vi "Try Match Response.vi"(8 "error in":errorcluster, 10 "ICAN CC Frame":refnum<class "ICAN CC Frame.lvclass">, 11 "Block Upload End Transfer in":refnum<class "Block Upload End Transfer.lvclass">) -> (0 "error out":errorcluster, 2 "Match":bool, 3 "SDO Transfer out":refnum<class "SDO Transfer.lvclass">)   [LabVIEW 2020, in "CANopen.lvlib" / "SDO Manager.lvlib" / "Block Upload End Transfer.lvclass"]
uses:
  Block Upload End Transfer.lvclass
  SDO Transfer/SDO Transfer.lvclass
  HAL/Source/Interfaces/ICAN CC Frame/ICAN CC Frame.lvclass
  Block Upload End Transfer.lvclass/Block Upload End Transfer.ctl
  CANopen Message/CANopen Message.lvclass
  SDO Transfer/SDO abort code.ctl
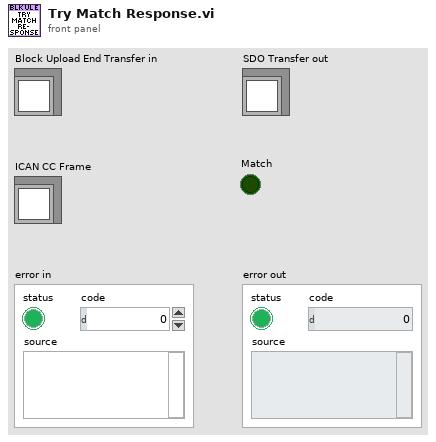
[diagram p1: front panel]
types:
  T1 = typedef "CANopen.lvlib/SDO Manager.lvlib/SDO Transfer.lvclass/SDO abort code.ctl" = u32
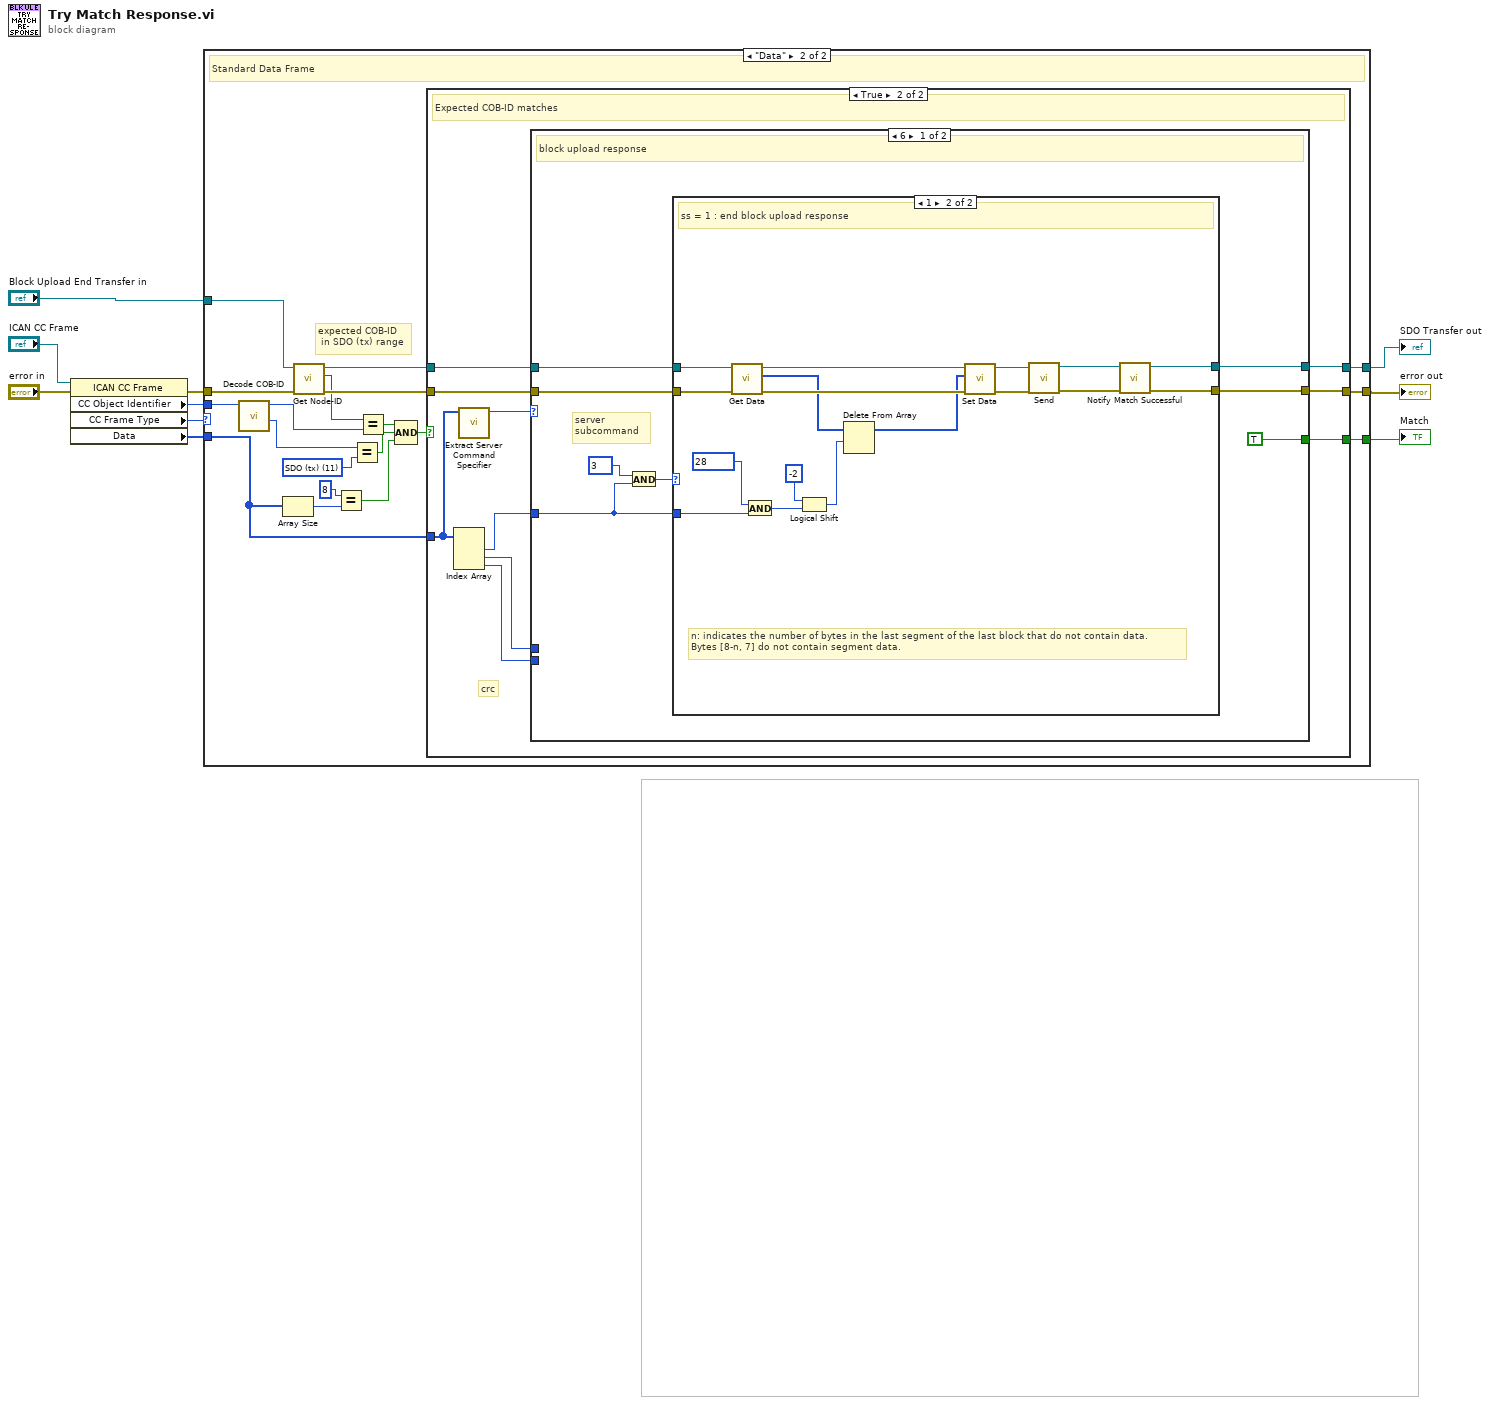
[diagram p0: block diagram]
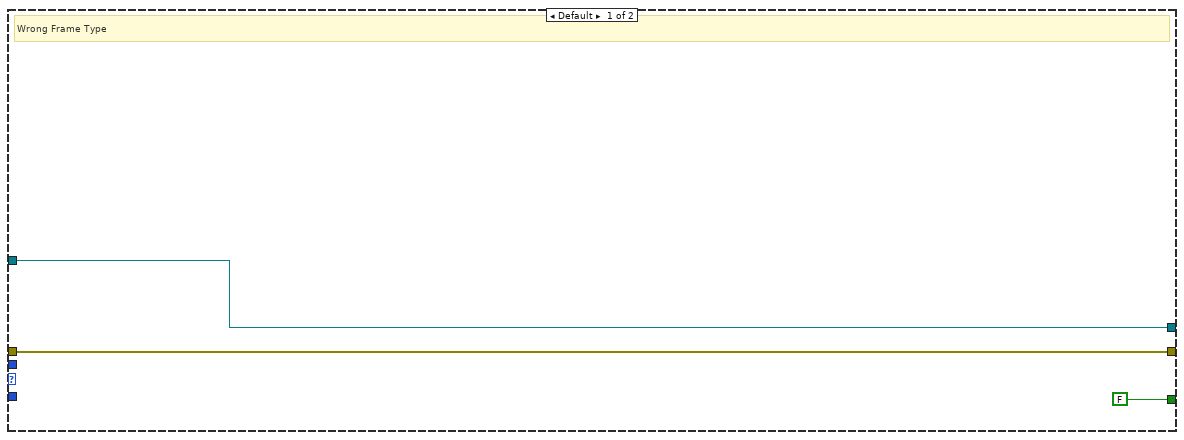
[diagram p2: hidden frame]
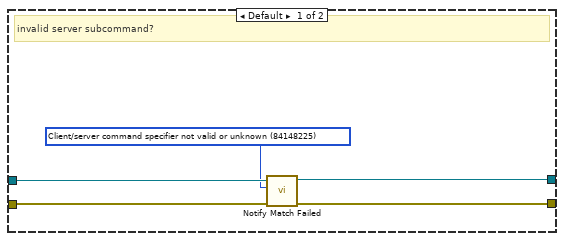
[diagram p4: hidden frame]
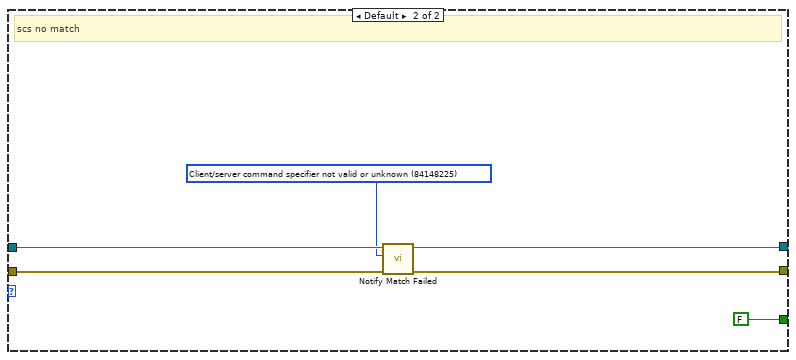
[diagram p5: hidden frame]
diagram:
  n1 = property class="ICAN CC Frame"(reference="ICAN CC Frame", error in="error in") -> (error out=w10:errorcluster, "CC Object Identifier"=w9:u32, "CC Frame Type"=w7:enum8{"Data", "Remote", "Error", "Overload"}, "Data"=w8:u8[])  [unwired: 1 out]
  n2 = case shown="\"Data\"" w7 {
    tunnel: w10 -> [w12 w32]
    tunnel: "Block Upload End Transfer in" -> [w11 w31]
    tunnel: [w11 w28] -> w4
    tunnel: [w12 w27] -> w6
    tunnel: [FALSE w26] -> w5
    tunnel: w9 -> [_ w25]
    tunnel: w8 -> [_ w14]
    frame Default {
      # "Wrong Frame Type"
    }
    frame "Data" {
      w22 = u8 11 items=["NMT"=0, "EMCY/SYNC"=1, "TIME"=2, "PDO1 (tx)"=3, "PDO1 (rx)"=4, "PDO2 (tx)"=5, "PDO2 (rx)"=6, "PDO3 (tx)"=7, "PDO3 (rx)"=8, "PDO4 (tx)"=9, "PDO4 (rx)"=10, "SDO (tx)"=11, "SDO (rx)"=12, "NMT error control"=14] ("Function Code")
      # "expected COB-ID\n in SDO (tx) range"
      # "Standard Data Frame"
      n3 = call "Decode COB-ID.vi"("COD-ID"=w25) -> ("Function Code"=w21:u8, "Node-ID"=w24:u8)  [unwired: 9 in]
      n4 = Array Size(array=w14) -> (size(s)=w20:i32)
      n5 = call "Get Node-ID.vi"("error in"=w32, "SDO Transfer in"=w31) -> ("error out"=w29:errorcluster, "Node-ID"=w23:u8, "SDO Transfer out"=w30:refnum<class "Block Upload End Transfer.lvclass">)  [unwired: 7 in]
      n6 = Equal?(x=8, y=w20) -> (x = y?=w15:bool)
      n7 = Equal?(x=w21, y=w22) -> (x = y?=w16:bool)
      n8 = Equal?(x=w23, y=w24) -> (x = y?=w17:bool)
      n9 = Compound Arithmetic op=AND(w17, w16, w15) -> (w18:bool)
      n10 = case shown="True" w18 {
        tunnel: w30 -> [w34 w44]
        tunnel: w29 -> [w33 w43]
        tunnel: [w34 w39] -> w28
        tunnel: [w33 w40] -> w27
        tunnel: w14 -> [_ w36]
        tunnel: [_ w38] -> w26
        frame False {
          # "no match"
        }
        frame True {
          # "crc"
          # "Expected COB-ID matches"
          n11 = Index Array(array=w36) -> (element #1=w37:u8, element #2=w42:u8, element #3=w41:u8)  [unwired: 3 in]
          n12 = call "Extract Server Command Specifier.vi"("Data"=w36) -> ("Server Command Specifier"=w35:u8)  [unwired: 10 in]
          n13 = case shown="6" w35 {
            tunnel: w42 -> [_ _]
            tunnel: w41 -> [_ _]
            tunnel: w44 -> [w49 w77]
            tunnel: w43 -> [w48 w80]
            tunnel: [w46 w76] -> w39
            tunnel: [w47 w78] -> w40
            tunnel: [TRUE FALSE] -> w38
            tunnel: w37 -> [w50 _]
            frame 6 {
              # "server\nsubcommand"
              # "block upload response"
              n14 = And(x=u8 3, y=w50) -> (x .and. y?=w51:u8)
              n15 = case shown="1" w51 {
                tunnel: w50 -> [_ w71]
                tunnel: w49 -> [w55 w69]
                tunnel: w48 -> [w57 w73]
                tunnel: [w56 w65] -> w47
                tunnel: [w54 w63] -> w46
                frame Default {
                  w53 = T1 84148225 items=["Toggle bit not allowed"=84082688, "SDO protocol timed out"=84148224, "Client/server command specifier not valid or unknown"=84148225, "Invalid block size (block mode only)"=84148226, "Invalid sequence number (block mode only)"=84148227, "CRC error (block mode only)"=84148228, "Out of memory"=84148229, "Attempt to read a write only object"=100728833, "Attempt to write a read only object"=100728834, "Object does not exist in the object dictionary"=100794368, "Object cannot be mapped to the PDO"=100925505, "The number and length of the objects to be mapped would exceed PDO length"=100925506, "General parameter incompatibility reason"=100925507, "General internal incompatibility in the device"=100925511, "Access failed due to an hardware error"=101056512, "Data type does not match, length of service parameter does not match"=101122064, "Data type does not match, length of service parameter too high"=101122066, "Data type does not match, length of service parameter too low"=101122067, "Sub-index does not exist"=101253137, "Invalid value for parameter (download only)"=101253168, "Value of parameter written too high (download only)"=101253169, "Value of parameter written too low (download only)"=101253170, "Maximum value is less than minimum value"=101253174, "Resource not available: SDO connection"=101318691, "General error"=134217728, "Data cannot be transferred or stored to the application"=134217760, "Data cannot be transferred or stored to the application because of local control"=134217761, "Data cannot be transferred or stored to the application because of the present device stable"=134217762, "Object dictionary dynamic generation fails or no object dictionary is present (e.g. object dictionary is generated from file and generation fails because of an file error)"=134217763, "No data available"=134217764] ("SDO abort code")
                  # "invalid server subcommand?"
                  n16 = call "Notify Match Failed.vi"("error in"=w57, "SDO abort code"=w53, "SDO Transfer in"=w55) -> ("error out"=w56:errorcluster, "SDO Transfer out"=w54:refnum<class "Block Upload End Transfer.lvclass">)  [unwired: 7 in]
                }
                frame 1 {
                  # "n: indicates the number of bytes in the last segment of the last block that do not contain data.\nBytes [8-n, 7] do not contain segment data."
                  # "ss = 1 : end block upload response"
                  n17 = call "Get Data.vi"("error in"=w73, "SDO Transfer in"=w69) -> ("error out"=w70:errorcluster, "Data"=w61:u8[], "SDO Transfer out"=w67:refnum<class "Block Upload End Transfer.lvclass">)  [unwired: 7 in]
                  n18 = And(x=u8 28, y=w71) -> (x .and. y?=w59:u8)
                  n19 = Logical Shift(y=i16 -2, x=w59) -> (x << y=w60:u8)
                  n20 = Delete From Array(array=w61, length=w60) -> (array with subset deleted=w62:u8[])  [unwired: 1 in, 1 out]
                  n21 = call "Set Data.vi"("error in"=w70, "Data"=w62, "SDO Transfer in"=w67) -> ("error out"=w68:errorcluster, "SDO Transfer out"=w66:refnum<class "Block Upload End Transfer.lvclass">)  [unwired: 7 in]
                  n22 = call-dynamic "Send.vi"("error in"=w68, "Block Upload End Transfer in"=w66) -> ("error out"=w74:errorcluster, "Block Upload End Transfer out"=w64:refnum<class "Block Upload End Transfer.lvclass">)  [unwired: 8 in]
                  n23 = call "Notify Match Successful.vi"("error in"=w74, "SDO Transfer in"=w64) -> ("error out"=w65:errorcluster, "SDO Transfer out"=w63:refnum<class "Block Upload End Transfer.lvclass">)  [unwired: 8 in]
                }
              }
            }
            frame Default {
              w75 = T1 84148225 items=["Toggle bit not allowed"=84082688, "SDO protocol timed out"=84148224, "Client/server command specifier not valid or unknown"=84148225, "Invalid block size (block mode only)"=84148226, "Invalid sequence number (block mode only)"=84148227, "CRC error (block mode only)"=84148228, "Out of memory"=84148229, "Attempt to read a write only object"=100728833, "Attempt to write a read only object"=100728834, "Object does not exist in the object dictionary"=100794368, "Object cannot be mapped to the PDO"=100925505, "The number and length of the objects to be mapped would exceed PDO length"=100925506, "General parameter incompatibility reason"=100925507, "General internal incompatibility in the device"=100925511, "Access failed due to an hardware error"=101056512, "Data type does not match, length of service parameter does not match"=101122064, "Data type does not match, length of service parameter too high"=101122066, "Data type does not match, length of service parameter too low"=101122067, "Sub-index does not exist"=101253137, "Invalid value for parameter (download only)"=101253168, "Value of parameter written too high (download only)"=101253169, "Value of parameter written too low (download only)"=101253170, "Maximum value is less than minimum value"=101253174, "Resource not available: SDO connection"=101318691, "General error"=134217728, "Data cannot be transferred or stored to the application"=134217760, "Data cannot be transferred or stored to the application because of local control"=134217761, "Data cannot be transferred or stored to the application because of the present device stable"=134217762, "Object dictionary dynamic generation fails or no object dictionary is present (e.g. object dictionary is generated from file and generation fails because of an file error)"=134217763, "No data available"=134217764] ("SDO abort code")
              # "scs no match"
              n24 = call "Notify Match Failed.vi"("error in"=w80, "SDO abort code"=w75, "SDO Transfer in"=w77) -> ("error out"=w78:errorcluster, "SDO Transfer out"=w76:refnum<class "Block Upload End Transfer.lvclass">)  [unwired: 7 in]
            }
          }
        }
      }
    }
  }
  "SDO Transfer out" <- w4
  "error out" <- w6
  "Match" <- w5
